vi "Sub02_PosTxt.vi"(8 "error in (no error) 2":errorcluster, 10 "input cluster":T1, 11 "working directory":path=path "") -> (0 "error out":errorcluster, 1 "resulting string":string, 3 "output cluster":T2, 5 "standard error":string, 7 "standard output":string)   [LabVIEW 2019]
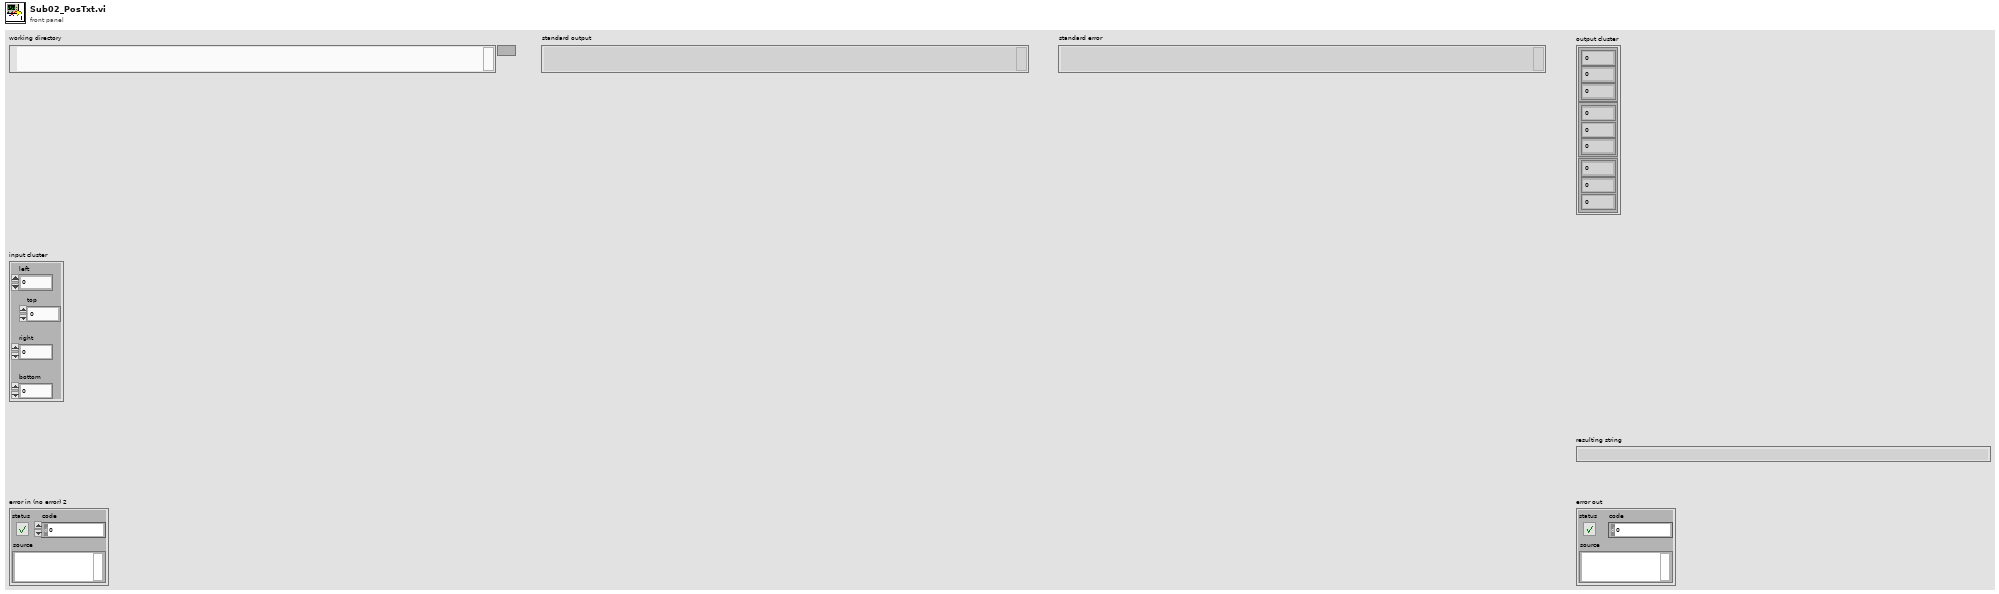
[diagram p1: front panel]
types:
  T1 = cluster{"left":u32, "top":u32, "right":u32, "bottom":u32}
  T2 = cluster{cluster{i32, i32, i32}, cluster{i32, i32, i32}, cluster{i32, i32, i32}}
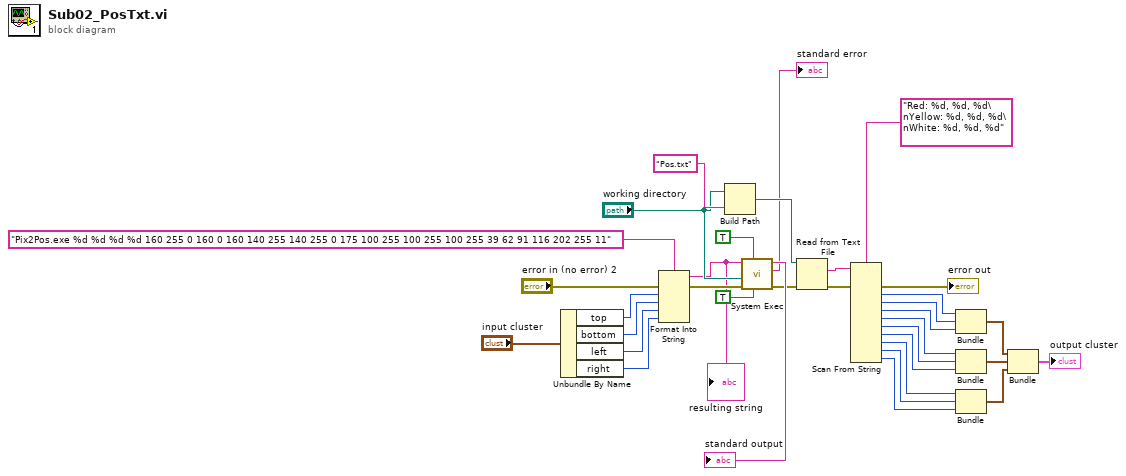
[diagram p0: block diagram]
diagram:
  n1 = Unbundle By Name("input cluster") -> ("top"=w7:u32, "bottom"=w6:u32, "left"=w5:u32, "right"=w4:u32)
  n2 = Format Into String(format string="Pix2Pos.exe %d %d %d %d 160 255 0 160 0 160 140 255 140 255 0 175 100 255 100 255 100 255 39 62 91 116 202 255 11", error in="error in (no error) 2", w7, w6, w5, w4) -> (resulting string=w1:string, error out=w2:errorcluster)  [unwired: 1 in]
  "resulting string" <- w1
  n3 = Build Path(base path="working directory", name or relative path="Pos.txt") -> (appended path=w31:path)
  n4 = call <vilib>:"System Exec.vi"("run minimized? (F)"=TRUE, "wait until completion? (T)"=TRUE, "error in (no error)"=w2, "working directory"="working directory", "command line"=w1) -> ("error out"=w10:errorcluster, "standard error"=→"standard error":string, "standard output"=→"standard output":string)  [unwired: 3 in, 1 out]
  n5 = Read from Text File(file (use dialog)=w31, error in=w10) -> (text=w33:string, error out=w30:errorcluster)  [unwired: 2 in, 2 out]
  n6 = Scan From String(format string="Red: %d, %d, %d\nYellow: %d, %d, %d\nWhite: %d, %d, %d", input string=w33, error in=w30) -> (error out=→"error out":errorcluster, output 1=w28:i32, output 2=w27:i32, output 3=w26:i32, output 4=w25:i32, output 5=w24:i32, output 6=w23:i32, output 7=w22:i32, output 8=w21:i32, output 9=w20:i32)  [unwired: 10 in, 2 out]
  n7 = Bundle(w28, w27, w26) -> (w19:cluster{i32, i32, i32})  [unwired: 1 in]
  n8 = Bundle(w25, w24, w23) -> (w18:cluster{i32, i32, i32})  [unwired: 1 in]
  n9 = Bundle(w22, w21, w20) -> (w17:cluster{i32, i32, i32})  [unwired: 1 in]
  n10 = Bundle(w19, w18, w17) -> (→"output cluster":T2)  [unwired: 1 in]
